vi "Fit VI window to Content.vi"(4 "error in (no error)":errorcluster, 6 "border spacing (2 px)":i32=2, 7 "VI Ref (calling VI)":refnum<vi>) -> (0 "error out":errorcluster, 3 "VI Ref out":refnum<vi>)   [LabVIEW 2017]
doc: "Resizes and centres the VI window around all front panel objects, adding the configured border spacing in pixels. With no VI reference wired it operates on the calling VI."
panel:
  # "Fit VI window to Content.vi\n\nFits a VI's front panel window to its FP Contents.\n\nPlease visit http://www.OpenG.org to learn about the\nOpen Source LabVIEW software movement.\n\nNOTICE -- YOU MUST LEAVE THIS NOTICE IN PLACE.  PER THE TERMS OF THE LICENSE BELOW, YOU MAY SUBLICENSE THIS SOFTWARE \nIN ANY WAY THAT DOES NOT CONFLICT WITH THIS LICENSE.\n\n### BSD License (http://www.opensource.org/licenses/bsd-license.php) Begin ###\n \nCopyright (c) 2002-2004, Jim Kring <jim@jimkring.com>\nCopyright (c) 2002, Cal-Bay Systems, Inc. <info@calbay.com>\n\nAll rights reserved.\n\nRedistribution and use in source and binary forms, with or without modification, are permitted provided that the following conditions are met:\n\n    * Redistributions of source code must retain the above copyright notice, this list of conditions and the following disclaimer.\n    * Redistributions in binary form must reproduce the above copyright notice, this list of conditions and the following disclaimer in the \n       documentation and/or other materials provided with the distribution.\n    * Neither the name of SciWare, James Kring, Inc., nor the names of its contributors may be used to endorse or promote products derived \n       from this software without specific prior written permission.\n\nTHIS SOFTWARE IS PROVIDED BY THE COPYRIGHT HOLDERS AND CONTRIBUTORS \"AS IS\" AND ANY EXPRESS OR IMPLIED WARRANTIES, \nINCLUDING, BUT NOT LIMITED TO, THE IMPLIED WARRANTIES OF MERCHANTABILITY AND FITNESS FOR A PARTICULAR PURPOSE ARE \nDISCLAIMED. IN NO EVENT SHALL THE COPYRIGHT OWNER OR CONTRIBUTORS BE LIABLE FOR ANY DIRECT, INDIRECT, INCIDENTAL,\n SPECIAL, EXEMPLARY, OR CONSEQUENTIAL DAMAGES (INCLUDING, BUT NOT LIMITED TO, PROCUREMENT OF SUBSTITUTE GOODS OR \nSERVICES; LOSS OF USE, DATA, OR PROFITS; OR BUSINESS INTERRUPTION) HOWEVER CAUSED AND ON ANY THEORY OF LIABILITY, \nWHETHER IN CONTRACT, STRICT LIABILITY, OR TORT (INCLUDING NEGLIGENCE OR OTHERWISE) ARISING IN ANY WAY OUT OF THE USE \nOF THIS SOFTWARE, EVEN IF ADVISED OF THE POSSIBILITY OF SUCH DAMAGE.\n\n### BSD License End ###"
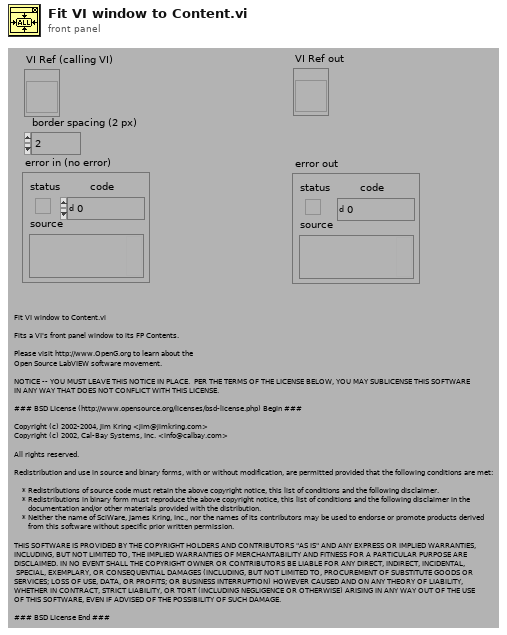
[diagram p1: front panel]
types:
  T1 = typedef "LVRectTypeDef.ctl" = cluster{"Left":i16, "Top":i16, "Right":i16, "Bottom":i16}
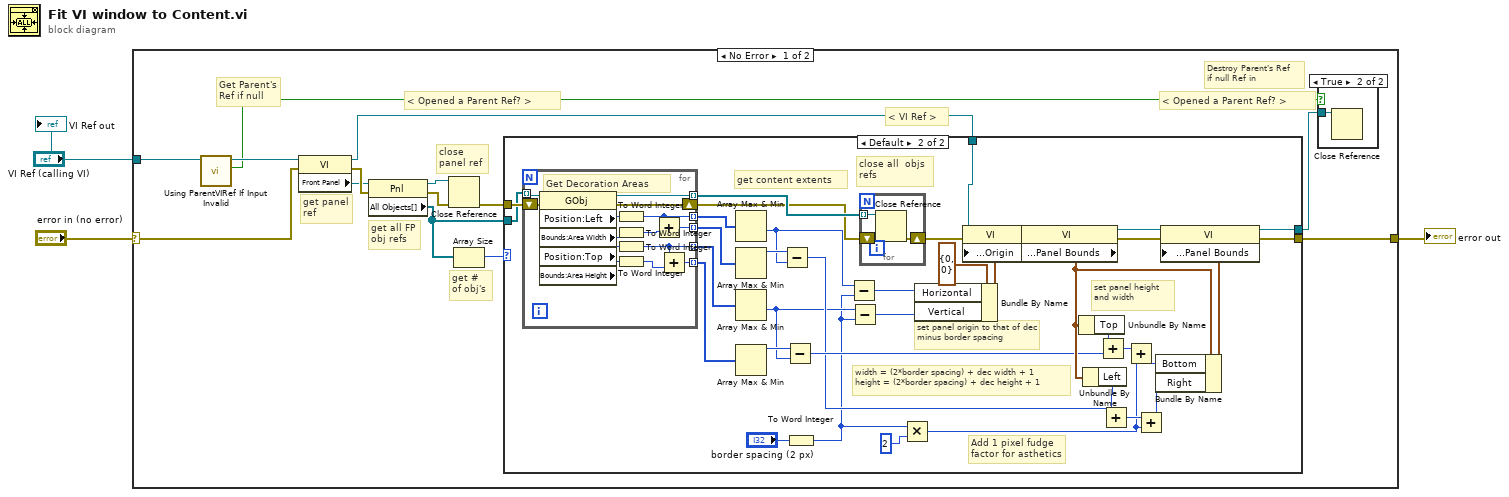
[diagram p0: block diagram]
diagram:
  n1 = case shown="No Error" "error in (no error)" {
    selector: "error in (no error)" -> [w6 w76]
    tunnel: [w11 w76] -> w3
    tunnel: "VI Ref (calling VI)" -> [w7 _]
    frame No Error {
      # "< Opened a Parent Ref? >"
      # "< Opened a Parent Ref? >"
      # "Destroy Parent's Ref\nif null Ref in"
      # "Get Parent's\nRef if null"
      # "get # of obj's"
      # "get panel ref"
      # "get all FP obj refs"
      # "close panel ref"
      # "< VI Ref >"
      n2 = call "Using ParentVIRef If Input Invalid.vi"("VI Ref (calling VI)"=w7) -> ("Using Parent Ref(Need to Destroy)"=w4:bool, "VI Ref"=w5:refnum<vi>)  [unwired: 5 in]
      n3 = property on="Property Node" class="VI"(reference=w5, error in=w6) -> (reference out=w17:refnum<vi>, error out=w15:errorcluster, "Front Panel"=w13:refnum<vi>)
      n4 = property on="Property Node" class="Pnl"(reference=w13, error in=w15) -> (reference out=w16:refnum<vi>, error out=w14:errorcluster, "All Objects[]"=w10:refnum<vi>[])
      n5 = Close Reference(reference=w16, error in (no error)=w14) -> (error out=w12:errorcluster)
      n6 = Array Size(array=w10) -> (size(s)=w9:i32)
      n7 = case shown="Default" w9 {
        tunnel: w17 -> [w20 w56]
        tunnel: w12 -> [w19 w43]
        tunnel: [w19 w38] -> w11
        tunnel: [w20 w37] -> w8
        tunnel: w10 -> [_ w36]
        frame 0 {
          # "do nothing if no objects"
        }
        frame Default {
          # "width = (2*border spacing) + dec width + 1\nheight = (2*border spacing) + dec height + 1"
          # "set panel height and width"
          # "set panel origin to that of dec minus border spacing"
          # "close all  objs refs"
          # "get content extents"
          # "Add 1 pixel fudge factor for asthetics"
          n8 = for {
            tunnel: w36 -> [w75] mode=indexing
            shift-right: [w73] -> w23
            shift-left: w43 -> [w74]
            tunnel: [w72] -> w24 mode=indexing
            tunnel: [w68] -> w34 mode=indexing
            tunnel: [w70] -> w33 mode=indexing
            tunnel: [w64] -> w32 mode=indexing
            tunnel: [w69] -> w31 mode=indexing
            # "Get Decoration Areas"
            n9 = property class="GObj"(reference=w75, error in=w74) -> (reference out=w72:refnum<vi>, error out=w73:errorcluster, "Position:Left"=w71:i32, "Bounds:Area Width"=w67:u32, "Position:Top"=w65:i32, "Bounds:Area Height"=w63:u32)
            n10 = To Word Integer(number=w71) -> (16bit integer=w68:i16)
            n11 = To Word Integer(number=w67) -> (16bit integer=w66:i16)
            n12 = To Word Integer(number=w65) -> (16bit integer=w64:i16)
            n13 = To Word Integer(number=w63) -> (16bit integer=w62:i16)
            n14 = Add(x=w68, y=w66) -> (x+y=w70:i16)
            n15 = Add(x=w64, y=w62) -> (x+y=w69:i16)
          }
          n16 = Array Max & Min(array=w34) -> (min value=w25:i16)  [unwired: 3 out]
          n17 = Array Max & Min(array=w33) -> (max value=w28:i16)  [unwired: 3 out]
          n18 = Array Max & Min(array=w32) -> (min value=w26:i16)  [unwired: 3 out]
          n19 = Array Max & Min(array=w31) -> (max value=w30:i16)  [unwired: 3 out]
          n20 = Subtract(x=w28, y=w25) -> (x-y=w27:i16)
          n21 = Subtract(x=w30, y=w26) -> (x-y=w29:i16)
          n22 = To Word Integer(number="border spacing (2 px)") -> (16bit integer=w21:i16)
          n23 = Subtract(x=w25, y=w21) -> (x-y=w46:i16)
          n24 = Subtract(x=w26, y=w21) -> (x-y=w47:i16)
          n25 = for {
            tunnel: w24 -> [w61] mode=indexing
            shift-right: [w59] -> w22
            shift-left: w23 -> [w60]
            n26 = Close Reference(reference=w61, error in (no error)=w60) -> (error out=w59:errorcluster)
          }
          n27 = Multiply(x=w21, y=i16 2) -> (x*y=w35:i16)
          n28 = Bundle By Name(cluster=cluster{"Horizontal":i16, "Vertical":i16} {"Horizontal"=0, "Vertical"=0} ("Front Panel Window:Origin"), "Horizontal"=w46, "Vertical"=w47) -> (w44:cluster{"Horizontal":i16, "Vertical":i16})
          n29 = property on="Property Node" class="VI"(reference=w56, error in=w22, "Front Panel Window:Origin"=w44) -> (reference out=w57:refnum<vi>, error out=w40:errorcluster)
          n30 = property on="Property Node" class="VI"(reference=w57, error in=w40) -> (reference out=w58:refnum<vi>, error out=w39:errorcluster, "Front Panel Window:Panel Bounds"=w48:T1)
          n31 = Unbundle By Name(w48) -> ("Top"=w49:i16)
          n32 = Unbundle By Name(w48) -> ("Left"=w50:i16)
          n33 = Add(x=w49, y=w29) -> (x+y=w54:i16)
          n34 = Add(x=w50, y=w27) -> (x+y=w52:i16)
          n35 = Add(x=w54, y=w35) -> (x+y=w55:i16)
          n36 = Add(x=w52, y=w35) -> (x+y=w53:i16)
          n37 = Bundle By Name(cluster=w48, "Bottom"=w55, "Right"=w53) -> (w51:T1)
          n38 = property on="Property Node" class="VI"(reference=w58, error in=w39, "Front Panel Window:Panel Bounds"=w51) -> (reference out=w37:refnum<vi>, error out=w38:errorcluster)
        }
      }
      n39 = case shown="True" w4 {
        tunnel: w8 -> [_ w18]
        frame False {
        }
        frame True {
          n40 = Close Reference(reference=w18) -> ()  [unwired: 1 in, 1 out]
        }
      }
    }
    frame Error {
    }
  }
  "error out" <- w3
  "VI Ref out" <- "VI Ref (calling VI)"
